vi "Run.vi"(8 "error in (no error)":errorcluster, 10 "Timing Source":string, 11 "Audio Output Queue":refnum<queue>) -> (0 "error out":errorcluster)   [LabVIEW 2019, in "Audio Engine.lvlib"]
doc: "The main audio processing loop.\n\n<b>Priority:</b> Above Normal\n<b>Execution System:</b> Standard"
uses:
  Audio Engine.lvlib
  Audio Output/Audio Output Queue Type.ctl
  <vilib>/Platform/TimedLoop/XDataNode/timing_clust.ctl
  <vilib>/Platform/TimedLoop/XDataNode/nitl_modes.ctl
  <vilib>/Platform/TimedLoop/XDataNode/wakeup.ctl
  Packed Libraries/Globals.lvlibp/Constants.vi
  Packed Libraries/Audio Processing.lvlibp/DBL To I16.vi
  <vilib>/platform/TimedLoop/XDataNode/XDataNode.xnode
  Classes/Deck/Deck.lvclass
  Classes/Mixer/Mixer.lvclass
  <vilib>/Platform/TimedLoop/XDataNode/XDNodeRunTimeDep.lvlib
  Audio Output/Audio Output.lvlib
  Packed Libraries/Globals.lvlibp
  Classes/Effect Unit/Effect Unit.lvclass
  Classes/Channel/Channel.lvclass
  Packed Libraries/Messaging.lvlibp
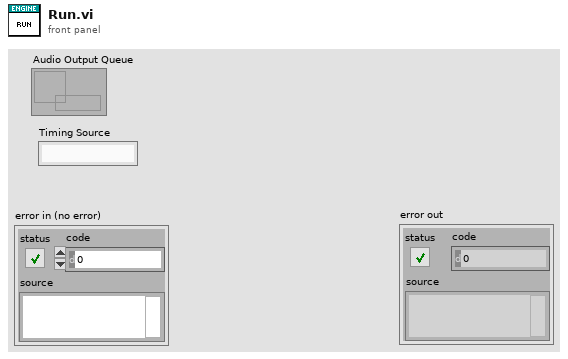
[diagram p1: front panel]
types:
  T1 = typedef "XDNodeRunTimeDep.lvlib/timing_clust.ctl" = cluster{"Expected End [f-1]":u64, "Actual End [f-1]":u64, "Finished Late? [f-1]":bool, "Expected End [i-1]":u64, "Actual End [i-1]":u64, "Finished Late? [i-1]":bool, "Expected Start [i]":u64, "Actual Start [i]":u64, "Expected Start [f]":u64, "Actual Start [f]":u64, "Source Name":string, "Structure Name":string, "Period":i64, "Deadline":i64, "Offset":i64, "Start":i64, "Priority":i32, "Timeout":i32, "Mode":T2, "Wakeup Reason":T3, "Error":errorcluster, "Source Type":string, "Secondary Source Type":string, "Global End Time":u64, "Global Start Time":u64, "Frame Duration":u64, "Iteration Duration":u64, "Assigned CPU":i32, "I/O Scan Engine Mode":u32}
  T2 = typedef "XDNodeRunTimeDep.lvlib/nitl_modes.ctl" = enum32{"No Change", "Process missed periods, maintain original phase", "Discard missed periods, maintain original phase", "Process missed periods, ignore original phase", "Discard missed periods, ignore original phase"}
  T3 = typedef "XDNodeRunTimeDep.lvlib/wakeup.ctl" = enum32{"Normal", "Aborted", "Asynchronous wakeup", "Timing source error", "Timed loop error", "Timeout"}
  T4 = typedef "Audio Output.lvlib/Audio Output Queue Type.ctl" = cluster{"Master":waveform(i16)[], "Headphones":waveform(i16)[], "Start Time":dbl}
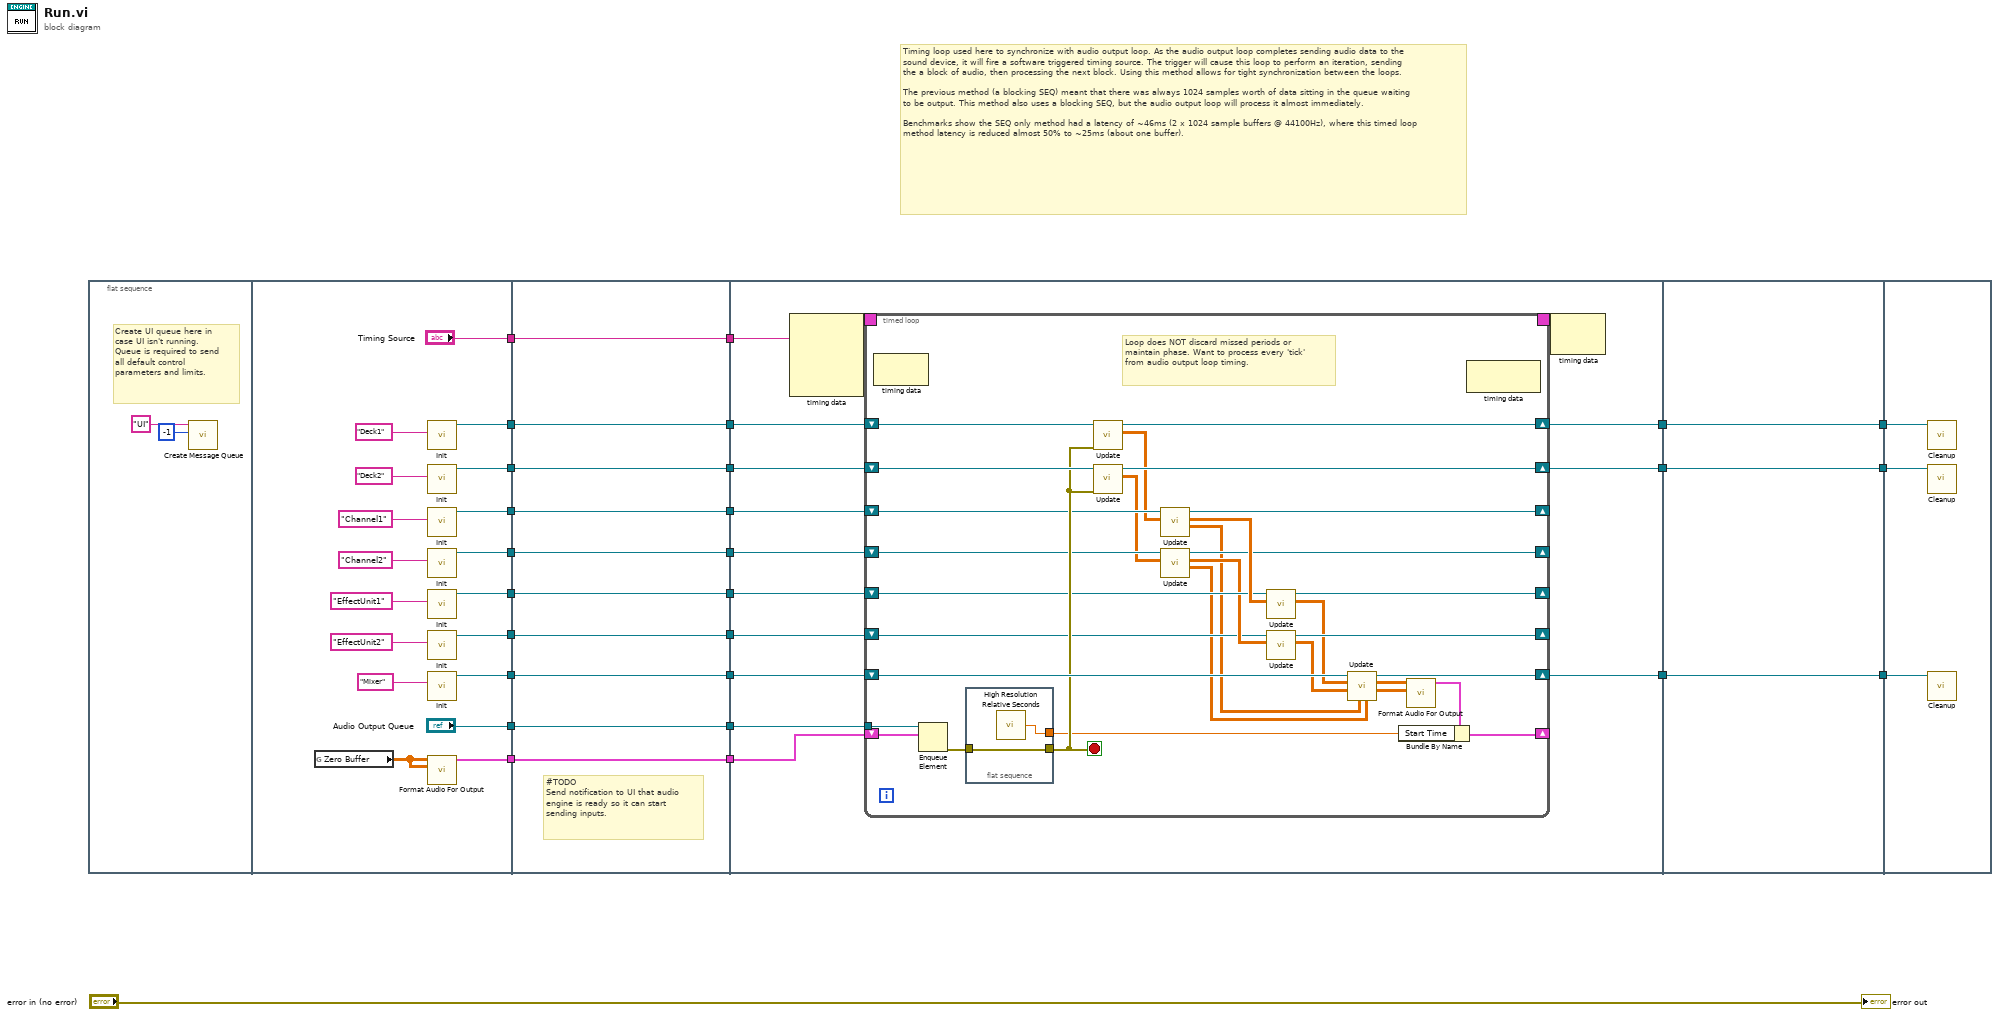
[diagram p0: block diagram]
diagram:
  # "Timing loop used here to synchronize with audio output loop. As the audio output loop completes sending audio data to the sound device, it will fire a software triggered timing source. The trigger will cause this loop to perform an iteration, sending the a block of audio, then processing the next block. Using this method allows for tight synchronization between the loops.\n\nThe previous method (a blocking SEQ) meant that there was always 1024 samples worth of data sitting in the queue waiting to be output. This method also uses a blocking SEQ, but the audio output loop will process it almost immediately.\n\nBenchmarks show the SEQ only method had a latency of ~46ms (2 x 1024 sample buffers @ 44100Hz), where this timed loop method latency is reduced almost 50% to ~25ms (about one buffer)."
  n1 = flat-sequence {
    tunnel: ["Audio Output Queue"] -> w26
    tunnel: [w43] -> w25
    tunnel: [w42] -> w24
    tunnel: [w41] -> w23
    tunnel: [w39] -> w11
    tunnel: ["Timing Source"] -> w9
    tunnel: [w35] -> w7
    tunnel: [w34] -> w5
    tunnel: [w31] -> w3
    tunnel: [w30] -> w1
    tunnel: w26 -> [w57]
    tunnel: w25 -> [w56]
    tunnel: w24 -> [w55]
    tunnel: w23 -> [w54]
    tunnel: [w57] -> w22
    tunnel: [w56] -> w21
    tunnel: [w55] -> w20
    tunnel: [w54] -> w19
    tunnel: [w53] -> w12
    tunnel: w11 -> [w53]
    tunnel: [w52] -> w10
    tunnel: w9 -> [w52]
    tunnel: [w51] -> w8
    tunnel: w7 -> [w51]
    tunnel: [w50] -> w6
    tunnel: w5 -> [w50]
    tunnel: [w49] -> w4
    tunnel: w3 -> [w49]
    tunnel: [w48] -> w2
    tunnel: w1 -> [w48]
    tunnel: w22 -> [w72]
    tunnel: w21 -> [w66]
    tunnel: w20 -> [w67]
    tunnel: w19 -> [w68]
    tunnel: [w71] -> w17
    tunnel: [w70] -> w15
    tunnel: [w69] -> w13
    tunnel: w12 -> [w63]
    tunnel: w10 -> [w62]
    tunnel: w8 -> [w61]
    tunnel: w6 -> [w60]
    tunnel: w4 -> [w59]
    tunnel: w2 -> [w58]
    tunnel: [w114] -> w18
    tunnel: w17 -> [w114]
    tunnel: [w113] -> w16
    tunnel: w15 -> [w113]
    tunnel: [w112] -> w14
    tunnel: w13 -> [w112]
    tunnel: w18 -> [w117]
    tunnel: w16 -> [w116]
    tunnel: w14 -> [w115]
    frame #0 {
      # "Create UI queue here in case UI isn't running. Queue is required to send all default control parameters and limits."
      n2 = call "Create Message Queue.vi"("Max Size (1000)"=-1, "Queue Name"="UI") -> ()  [unwired: 8 in, 2 out]
    }
    frame #1 {
      n3 = global read "Constants.vi" "Zero Buffer"() -> (w40:dbl[][])
      n4 = call "Init.vi"("ID"="Deck1") -> ("Deck out"=w43:refnum<class "Deck.lvclass">)  [unwired: 9 in, 1 out]
      n5 = call "Init.vi"("ID"="Deck2") -> ("Deck out"=w42:refnum<class "Deck.lvclass">)  [unwired: 9 in, 1 out]
      n6 = call "Init.vi"("ID"="Channel1") -> ("Channel out"=w31:refnum<class "Channel.lvclass">)  [unwired: 9 in, 1 out]
      n7 = call "Init.vi"("ID"="Channel2") -> ("Channel out"=w30:refnum<class "Channel.lvclass">)  [unwired: 9 in, 1 out]
      n8 = call "Init.vi"("ID"="EffectUnit1") -> ("Effect Unit out"=w35:refnum<class "Effect Unit.lvclass">)  [unwired: 9 in, 1 out]
      n9 = call "Init.vi"("ID"="EffectUnit2") -> ("Effect Unit out"=w34:refnum<class "Effect Unit.lvclass">)  [unwired: 9 in, 1 out]
      n10 = call "Init.vi"("ID"="Mixer") -> ("Mixer out"=w41:refnum<class "Mixer.lvclass">)  [unwired: 9 in, 1 out]
      n11 = call "Format Audio For Output.vi"("Headphone Audio"=w40, "Master Audio"=w40) -> ("Audio Output"=w39:T4)  [unwired: 9 in]
    }
    frame #2 {
      # "#TODO\nSend notification to UI that audio engine is ready so it can start sending inputs."
    }
    frame #3 {
      n12 = node-c288(w62) -> (w65:T1)  [unwired: 3 in]
      n13 = timed-loop {
        shift-right: [w102] -> w71
        shift-left: w66 -> [w103]
        tunnel: w72 -> [w101]
        shift-right: [w99] -> w70
        shift-left: w67 -> [w100]
        shift-right: [w97] -> w69
        shift-left: w68 -> [w98]
        timing: w65 -> [_]
        timing-out: [_] -> w64
        shift-right: [w89] -> _
        shift-left: w63 -> [w94]
        shift-right: [w77] -> _
        shift-left: w61 -> [w81]
        shift-right: [w78] -> _
        shift-left: w60 -> [w79]
        shift-right: [w83] -> _
        shift-left: w59 -> [w88]
        shift-right: [w82] -> _
        shift-left: w58 -> [w87]
        stop <- w93 stop-if-true
        # "Loop does NOT discard missed periods or maintain phase. Want to process every 'tick' from audio output loop timing."
        n14 = node-c288() -> ()  [unwired: 1 in, 1 out]
        n15 = Enqueue Element(queue=w101, element=w94) -> (error out=w92:errorcluster)  [unwired: 2 in, 2 out]
        n16 = flat-sequence {
          tunnel: [w105] -> w93
          tunnel: w92 -> [w105]
          tunnel: [w104] -> w91
          frame #0 {
            n17 = call <vilib>:"High Resolution Relative Seconds.vi"() -> ("relative seconds"=w104:dbl)
          }
        }
        n18 = call "Update.vi"("error in (no error)"=w93, "Deck in"=w103) -> ("Audio Block"=w86:dbl[][], "Deck out"=w102:refnum<class "Deck.lvclass">)  [unwired: 7 in, 1 out]
        n19 = call "Update.vi"("error in (no error)"=w93, "Deck in"=w100) -> ("Audio Block"=w85:dbl[][], "Deck out"=w99:refnum<class "Deck.lvclass">)  [unwired: 7 in, 1 out]
        n20 = call "Update.vi"("Audio Block In"=w86, "Channel in"=w88) -> ("Headphones Audio Block Out"=w74:dbl[][], "Master Audio Block Out"=w84:dbl[][], "Channel out"=w83:refnum<class "Channel.lvclass">)  [unwired: 6 in, 1 out]
        n21 = call "Update.vi"("Audio Block In"=w85, "Channel in"=w87) -> ("Headphones Audio Block Out"=w73:dbl[][], "Master Audio Block Out"=w80:dbl[][], "Channel out"=w82:refnum<class "Channel.lvclass">)  [unwired: 6 in, 1 out]
        n22 = call "Update.vi"("Audio Block In"=w84, "Effect Unit in"=w81) -> ("Audio Block Out"=w76:dbl[][], "Effect Unit out"=w77:refnum<class "Effect Unit.lvclass">)  [unwired: 7 in, 1 out]
        n23 = call "Update.vi"("Audio Block In"=w80, "Effect Unit in"=w79) -> ("Audio Block Out"=w75:dbl[][], "Effect Unit out"=w78:refnum<class "Effect Unit.lvclass">)  [unwired: 7 in, 1 out]
        n24 = call "Update.vi"("Headphone Block 2"=w73, "Headphone Block 1"=w74, "Audio Block 2"=w75, "Audio Block 1"=w76, "Mixer in"=w98) -> ("Headphones Audio Block Out"=w95:dbl[][], "Master Audio Block Out"=w96:dbl[][], "Mixer out"=w97:refnum<class "Mixer.lvclass">)  [unwired: 3 in, 1 out]
        n25 = call "Format Audio For Output.vi"("Headphone Audio"=w95, "Master Audio"=w96) -> ("Audio Output"=w90:T4)  [unwired: 9 in]
        n26 = Bundle By Name(cluster=w90, "Start Time"=w91) -> (w89:T4)
        n27 = node-c288() -> ()  [unwired: 1 in, 1 out]
      }
      n28 = node-c288(w64) -> ()  [unwired: 1 out]
    }
    frame #4 {
    }
    frame #5 {
      n29 = call "Cleanup.vi"("Deck in"=w117) -> ()  [unwired: 9 in, 2 out]
      n30 = call "Cleanup.vi"("Deck in"=w116) -> ()  [unwired: 9 in, 2 out]
      n31 = call "Cleanup.vi"("Mixer in"=w115) -> ()  [unwired: 10 in, 1 out]
    }
  }
  "error out" <- "error in (no error)"
